vi "extract From Input Packet ENC Vel.vi"(10 "channel":i32, 11 "instance":i32) -> (3 "function return":i16)   [LabVIEW 2025, in "SADI_FW3.lvlib"]
doc: "SADI_API_Wrapper int16_t extractFromInputPacket_ENCVel(int instance,int channel);\nSADI_API_Wrapper uint16_t extractFromInputPacket_ENCVel(int instance,int channel);"
uses:
  SADI_FW3.lvlib
  SADI_FW3.dll
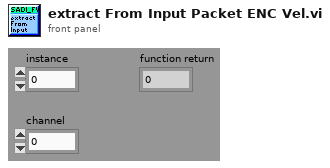
[diagram p1: front panel]
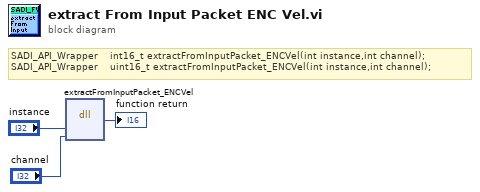
[diagram p0: block diagram]
diagram:
  # "SADI_API_Wrapper    int16_t extractFromInputPacket_ENCVel(int instance,int channel);\nSADI_API_Wrapper    uint16_t extractFromInputPacket_ENCVel(int instance,int channel);"
  n1 = dll-call lib="C:/Users/noaht/iCloudDrive/#1 School/Fall 2025/Controls Lab/LabView/EML4314c_FA25_framework_0/LVLib/SADI_FW3.*" fn="extractFromInputPacket_ENCVel"("instance"="instance", "channel"="channel") -> ("return type"=→"function return":i16)  [unwired: 5 in, 2 out]
